vi "TxP Fetch.vi"(7 "Selector String":string, 8 "error in (no error)":errorcluster, 11 "Instrument Handle In":refnum<k21>) -> (0 "error out":errorcluster, 2 "TxP Results":T1 {"Minimum Power (dBm)" format="%.2f"; "Maximum Power (dBm)" format="%.2f"; "Peak to Average Ratio (dB)" format="%.2f"; "Average Mean Power (dBm)" format="%.2f"}, 3 "Instrument Handle Out":refnum<k21>)   [LabVIEW 2016, in "RFmxSpecAn.lvlib"]
uses:
  RFmxSpecAn.lvlib
  Typedefs/TxP Results.ctl
  <vilib>/RFmx/SpecAn/mx/RFmxSpecAn.llb/RFmxSpecAn TXP Fetch Power Trace.vi
  <vilib>/RFmx/SpecAn/mx/RFmxSpecAn.llb/RFmxSpecAn TXP Fetch Measurement.vi
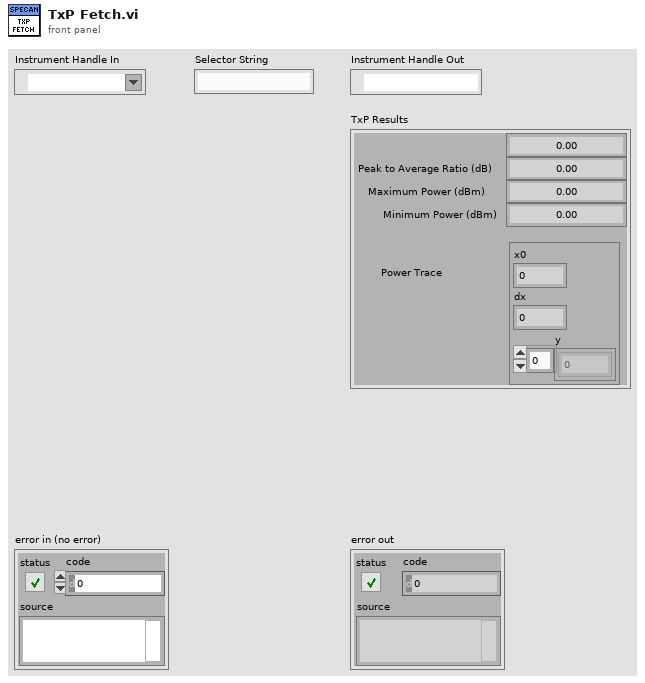
[diagram p1: front panel]
types:
  T1 = typedef "RFmxSpecAn.lvlib/TxP Results.ctl" = cluster{"Average Mean Power (dBm)":dbl, "Peak to Average Ratio (dB)":dbl, "Maximum Power (dBm)":dbl, "Minimum Power (dBm)":dbl, "Power Trace":cluster{"x0":dbl, "dx":dbl, "y":sgl[]}}
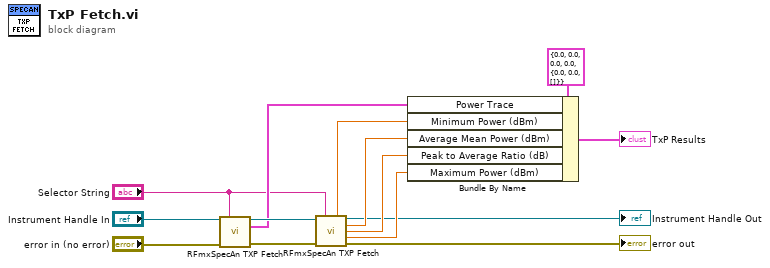
[diagram p0: block diagram]
diagram:
  n1 = call-poly <vilib>:"RFmxSpecAn TXP Fetch.vi"("Instrument Handle In"="Instrument Handle In", "Selector String"="Selector String", "error in (no error)"="error in (no error)") -> ("Instrument Handle Out"=w14:refnum<k21>, "Power (dBm)"=w11:cluster{"x0":dbl, "dx":dbl, "y":sgl[]}, "error out"=w13:errorcluster)  [unwired: 10 in]
  n2 = call-poly <vilib>:"RFmxSpecAn TXP Fetch.vi"("Instrument Handle In"=w14, "Selector String"="Selector String", "error in (no error)"=w13) -> ("Minimum Power (dBm)"=w7:dbl, "Instrument Handle Out"=→"Instrument Handle Out":refnum<k21>, "Average Mean Power (dBm)"=w10:dbl, "Peak to Average Ratio (dB)"=w9:dbl, "Maximum Power (dBm)"=w8:dbl, "error out"=→"error out":errorcluster)  [unwired: 7 in]
  n3 = Bundle By Name(cluster=T1 {"Average Mean Power (dBm)"=0.0, "Peak to Average Ratio (dB)"=0.0, "Maximum Power (dBm)"=0.0, "Minimum Power (dBm)"=0.0, "Power Trace"={"x0"=0.0, "dx"=0.0, "y"=[]}} ("Cluster"), "Power Trace"=w11, "Minimum Power (dBm)"=w7, "Average Mean Power (dBm)"=w10, "Peak to Average Ratio (dB)"=w9, "Maximum Power (dBm)"=w8) -> (→"TxP Results":T1)
